vi "Find max correlation.vi"() -> ()   [LabVIEW 2022 SP3]
uses:
  Globals/Meas_global.vi
panel:
  out "Delay index":i32
  out "Max Cross Correlation":dbl
  in  "Averaging period (ms)":dbl=500.0
  out "With Delay Shift":T1(graph)
  out "Cross Correlation":T2(graph)
  out "Not delay shift":T1(graph)
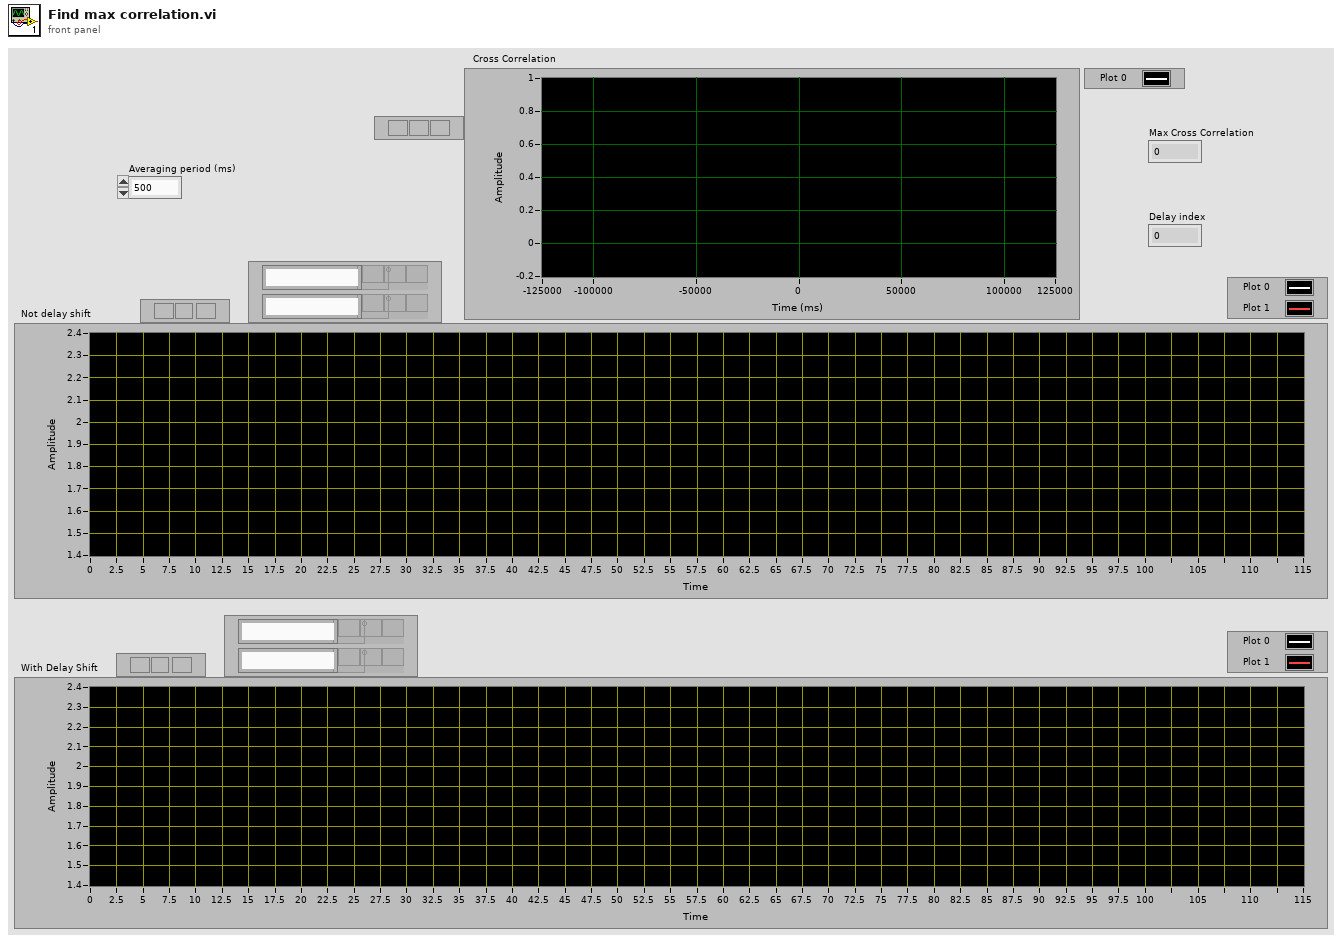
[diagram p1: front panel]
types:
  T1 = cluster{"Centre Time (s)":dbl[], "Eng Values 2":dbl[]}[]
  T2 = cluster{dbl, "Averaging period (ms)":dbl, "Cross Correlation":dbl[]}
  T3 = typedef "Time_Trace_Cluster.ctl" = cluster{"Weighting":dbl[], "Voltage":dbl[], "Eng Values":dbl[]}
  T4 = cluster{"Centre Time (s)":dbl[], "Eng Values 1":dbl[]}
  T5 = cluster{"Centre Time (s)":dbl[], "Eng Values 2":dbl[]}
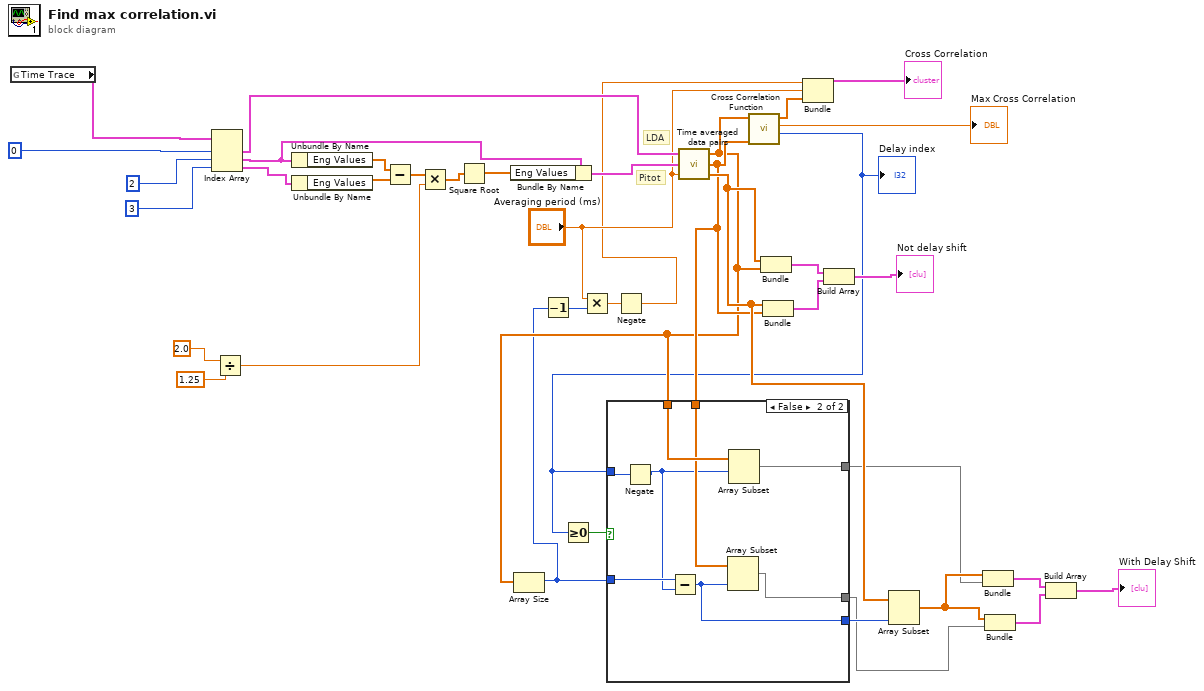
[diagram p0: block diagram]
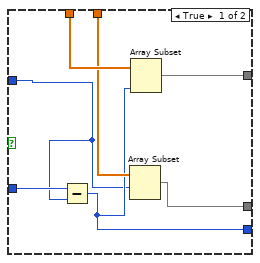
[diagram p2: hidden frame]
diagram:
  # "Pitot"
  # "LDA"
  n1 = global read "Meas_global.vi" "Time Trace"() -> (w38:T3[])
  n2 = Index Array(array=w38, index #1=0 ("index"), index #2=2 ("index"), index #3=3 ("index")) -> (element #1=w30:T3, element #2=w32:T3, element #3=w35:T3)
  n3 = Divide(x=2.0, y=1.25) -> (x/y=w22:dbl)
  n4 = Unbundle By Name(w32) -> ("Eng Values"=w34:dbl[])
  n5 = Unbundle By Name(w35) -> ("Eng Values"=w33:dbl[])
  n6 = Subtract(x=w34, y=w33) -> (x-y=w23:dbl[])
  n7 = Multiply(x=w23, y=w22) -> (x*y=w21:dbl[])
  n8 = Square Root(x=w21) -> (sqrt(x)=w26:dbl[])
  n9 = Bundle By Name(cluster=w32, "Eng Values"=w26) -> (w31:T3)
  n10 = call "Time averaged data pairs.vi"("Averaging period (ms)"="Averaging period (ms)", "Time Cluster 2"=w31, "Time Cluster 1"=w30) -> ("Centre Time (s)"=w15:dbl[], "Eng Values 2"=w11:dbl[], "Eng Values 1"=w10:dbl[])
  n11 = Array Size(array=w10) -> (size(s)=w2:i32)
  n12 = Decrement(x=w2) -> (x-1=w1:i32)
  n13 = Multiply(x="Averaging period (ms)", y=w1) -> (x*y=w4:dbl)
  n14 = Negate(x=w4) -> (-x=w3:dbl)
  n15 = call "Cross Correlation Function.vi"("Eng Values 2"=w11, "Eng Values 1"=w10) -> ("Delay index"=w9:i32, "Max Cross Correlation"=→"Max Cross Correlation":dbl, "Cross Correlation"=w7:dbl[])  [unwired: 2 in, 1 out]
  "Delay index" <- w9
  n16 = Greater Or Equal To 0?(x=w9) -> (x >= 0?=w17:bool)
  n17 = case shown="False" w17 {
    tunnel: w9 -> [w40 w48]
    tunnel: w10 -> [w46 w54]
    tunnel: w11 -> [w45 w53]
    tunnel: w2 -> [w44 w52]
    tunnel: [w41 w51] -> w16
    tunnel: [w43 w50] -> w13
    tunnel: [w42 w49] -> w12
    frame True {
      n18 = Subtract(x=w44, y=w40) -> (x-y=w41:i32)
      n19 = Array Subset(array=w45, index=w40) -> (w42:dbl[])  [unwired: 1 in]
      n20 = Array Subset(array=w46, length=w41) -> (w43:dbl[])  [unwired: 1 in]
    }
    frame False {
      n21 = Negate(x=w48) -> (-x=w47:i32)
      n22 = Subtract(x=w52, y=w47) -> (x-y=w51:i32)
      n23 = Array Subset(array=w53, length=w51) -> (w49:dbl[])  [unwired: 1 in]
      n24 = Array Subset(array=w54, index=w47) -> (w50:dbl[])  [unwired: 1 in]
    }
  }
  n25 = Bundle("Centre Time (s)"=w15, "Eng Values 1"=w10) -> (w28:T4)  [unwired: 1 in]
  n26 = Bundle("Centre Time (s)"=w15, "Eng Values 2"=w11) -> (w29:T5)  [unwired: 1 in]
  n27 = Bundle(w3, "Averaging period (ms)"="Averaging period (ms)", "Cross Correlation"=w7) -> (→"Cross Correlation":T2)  [unwired: 1 in]
  n28 = Build Array(w28, w29) -> (→"Not delay shift":T1)
  n29 = Array Subset(array=w15, length=w16) -> (w14:dbl[])  [unwired: 1 in]
  n30 = Bundle(w14, w13) -> (w18:cluster{dbl[], dbl[]})  [unwired: 1 in]
  n31 = Bundle(w14, w12) -> (w19:cluster{dbl[], dbl[]})  [unwired: 1 in]
  n32 = Build Array(w18, w19) -> (→"With Delay Shift":cluster{dbl[], dbl[]}[])
